vi "Test File Read.vi"() -> ()   [LabVIEW 2012]
uses:
  Controls/crd_data_enum.ctl
panel:
  out "data 2":sgl[][](array[numeric])
  out "data":sgl[](array[numeric])
  out "Array":timestamp[](array[timestamp])
  out "error out":errorcluster
  out "Numeric":i32
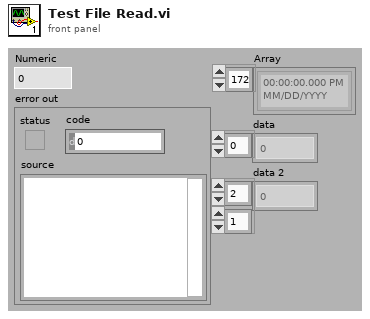
[diagram p1: front panel]
types:
  T1 = typedef "cPAS Library.lvlib/crd_data_enum.ctl" = enum8{"Time", "RHw", "TRH", "P", "Tmean", "RHsense", "TQ", "PQ", "Q", "Q0", "Qcal", "Qset", "extDilFac", "taucorr", "tau0corr", "stdevtau", "ext", "extCorr", "etau", "tau", "tau0", "Purge_Data", "NoData", "reserved", "Ttec", "Ang Exp", "Gamma", "filter", "fOverride", "notes", "max amp", "Tthermistor", "RhdilFac", "Psense", "TRHsense_bank", "RHsense_bank", "MFC_Data", "Thum", "ThumSP"}
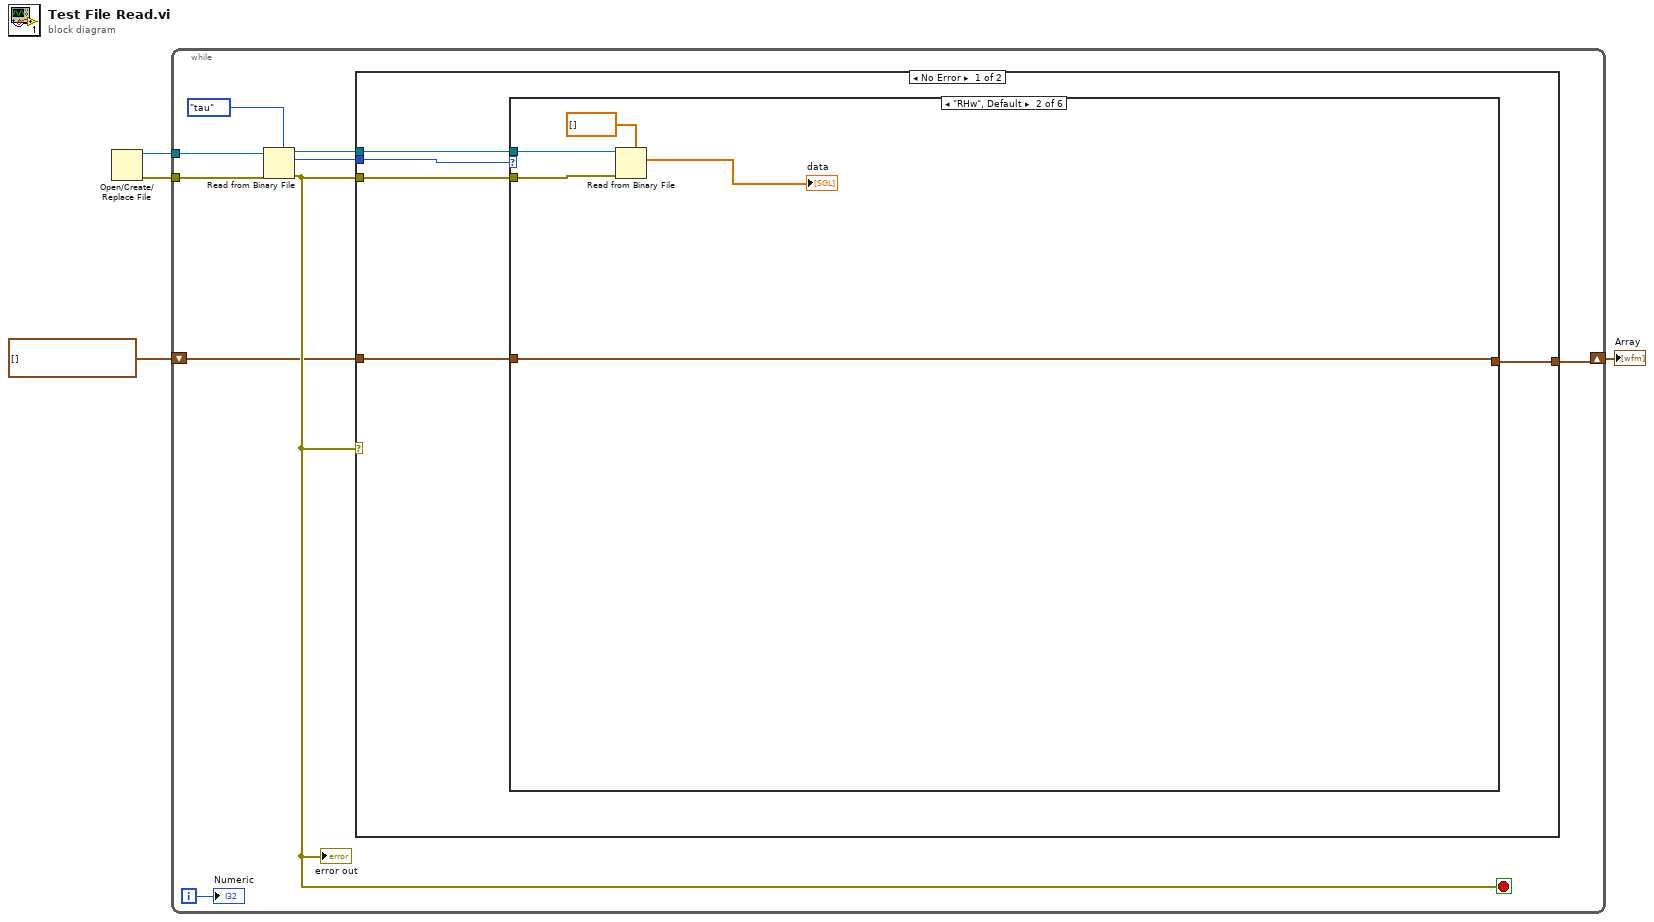
[diagram p0: block diagram]
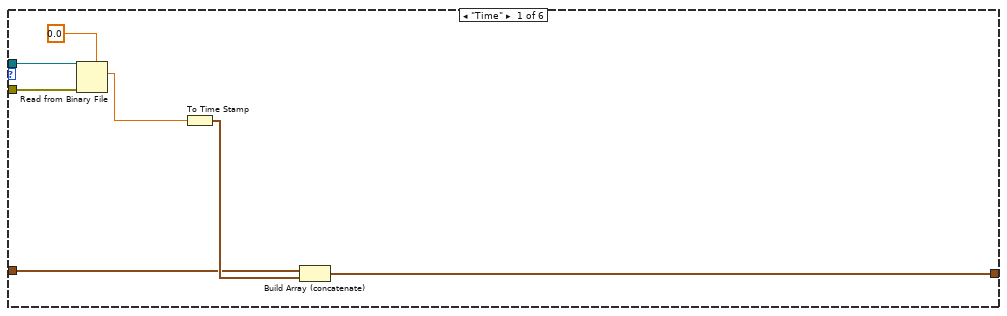
[diagram p2: hidden frame]
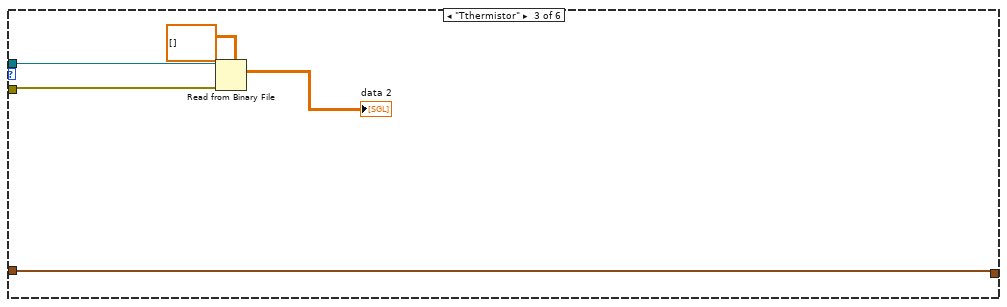
[diagram p3: hidden frame]
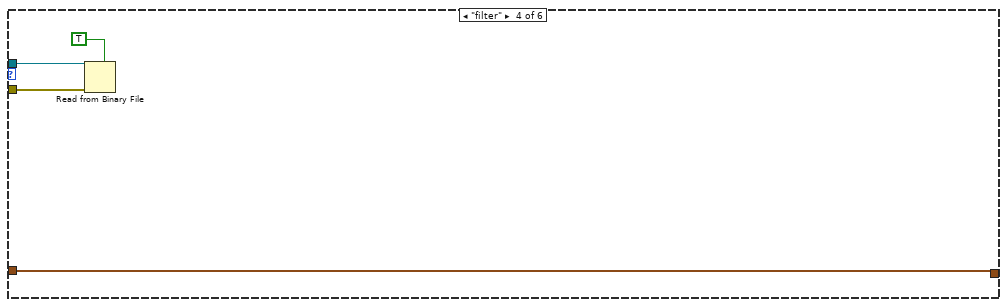
[diagram p4: hidden frame]
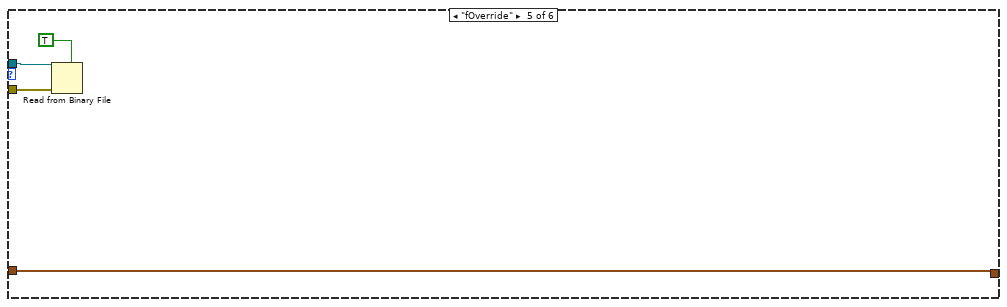
[diagram p5: hidden frame]
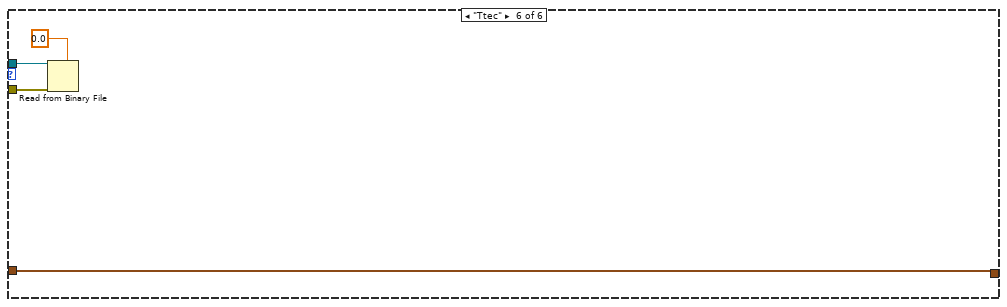
[diagram p6: hidden frame]
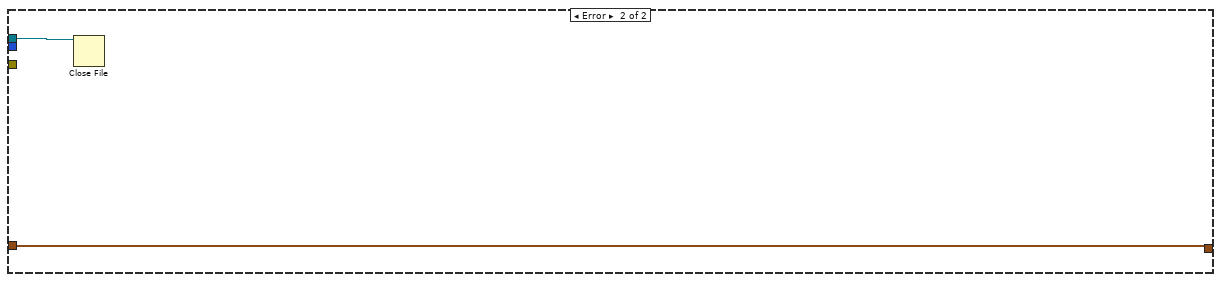
[diagram p7: hidden frame]
diagram:
  n1 = Open/Create/Replace File() -> (refnum out=w4:refnum<file>, error out=w3:errorcluster)  [unwired: 6 in, 1 out]
  n2 = while {
    tunnel: w4 -> [w13]
    tunnel: w3 -> [w12]
    shift-right: [w5] -> w1
    shift-left: timestamp[] [] -> [w6]
    i -> [w7]
    stop <- w9 stop-if-true
    n3 = Read from Binary File(5:crd_data_enum."tau" ("CRD_Data_Enum"), 8:w12, 11:w13) -> (0:w9:errorcluster, 2:w8:T1, 3:w10:refnum<file>)  [unwired: 3 in, 1 out]
    "error out" <- w9
    n4 = case shown="No Error" w9 {
      tunnel: w10 -> [w17 w49]
      tunnel: w9 -> [w16 _]
      tunnel: w8 -> [w18 _]
      tunnel: w6 -> [w15 w48]
      tunnel: [w14 w48] -> w5
      frame No Error {
        n5 = case shown="\"RHw\", Default" w18 {
          tunnel: w17 -> [w25 w29 w34 w38 w43 w46]
          tunnel: w16 -> [w24 w28 w33 w37 w41 w45]
          tunnel: w15 -> [w20 w27 w32 w36 w40 w47]
          tunnel: [w19 w27 w32 w36 w40 w47] -> w14
          frame "Time" {
            n6 = Read from Binary File(5:0.0, 8:w24, 11:w25) -> (2:w22:dbl)  [unwired: 3 in, 3 out]
            n7 = To Time Stamp(1:w22) -> (0:w21:timestamp)
            n8 = Build Array (concatenate)(w20, w21) -> (w19:timestamp[])
          }
          frame "RHw", Default {
            n9 = Read from Binary File(5:sgl[] [], 8:w28, 11:w29) -> (2:→"data":sgl[])  [unwired: 3 in, 3 out]
          }
          frame "Tthermistor" {
            n10 = Read from Binary File(5:sgl[][] [], 8:w33, 11:w34) -> (2:→"data 2":sgl[][])  [unwired: 3 in, 3 out]
          }
          frame "filter" {
            n11 = Read from Binary File(5:TRUE, 8:w37, 11:w38) -> ()  [unwired: 3 in, 4 out]
          }
          frame "fOverride" {
            n12 = Read from Binary File(5:TRUE, 8:w41, 11:w43) -> ()  [unwired: 3 in, 4 out]
          }
          frame "Ttec" {
            n13 = Read from Binary File(5:sgl 0.0, 8:w45, 11:w46) -> ()  [unwired: 3 in, 4 out]
          }
        }
      }
      frame Error {
        n14 = Close File(refnum=w49) -> ()  [unwired: 1 in, 2 out]
      }
    }
    "Numeric" <- w7
  }
  "Array" <- w1
